vi "NI VeriStand - Search for Item by Property.vi"(8 "error in":errorcluster, 9 "Property Value":variant, 10 "Property Name":string, 11 "Section Ref in":T1 format="%.0x") -> (0 "error out":errorcluster, 2 "Item Ref":T1 format="%.0x", 3 "Section Ref out":T1 format="%.0x", 4 "Found":bool)   [LabVIEW 2020, in "Custom Device Utility Library.lvlib"]
doc: "Searches a custom device section for the item(s) you specify. You can search for one or multiple items by name, GUID, or property name and value. You must manually select the polymorphic instance to use."
uses:
  <vilib>/NI VeriStand/Custom Device Tools/Custom Device Utility Library/Custom Device Utility Library.lvlib
  <vilib>/NI VeriStand/Custom Device API/Custom Device Item Ref.ctl
  <vilib>/NI VeriStand/Custom Device Tools/Custom Device Utility Library/NI VeriStand - Ref Constants.vi
  <vilib>/NI VeriStand/Custom Device API/Get Item Property (Variant).vi
  <vilib>/NI VeriStand/Custom Device API/Custom Device API.lvlib
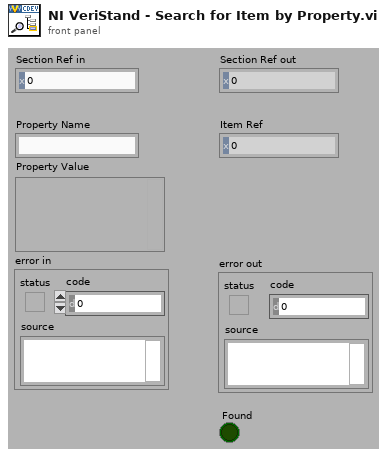
[diagram p1: front panel]
types:
  T1 = typedef "Custom Device API.lvlib/Custom Device Item Ref.ctl" = u64
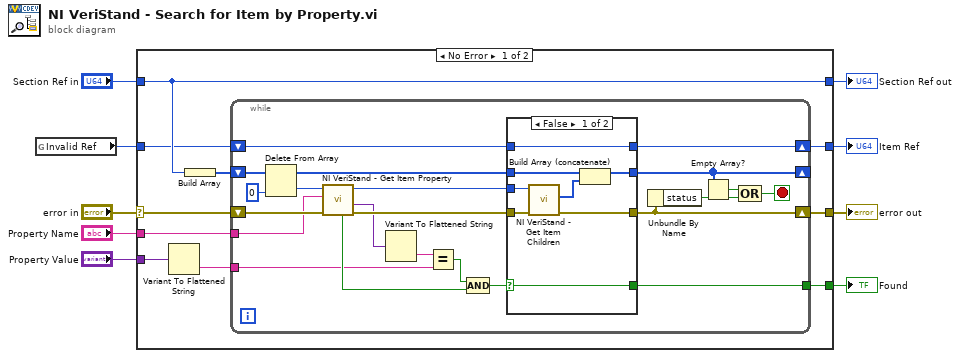
[diagram p0: block diagram]
diagram:
  n1 = global read "NI VeriStand - Ref Constants.vi" "Invalid Ref"() -> (w2:T1)
  n2 = case shown="No Error" "error in" {
    selector: "error in" -> [w14 w54]
    tunnel: "Section Ref in" -> [w15 w55]
    tunnel: "Property Name" -> [w18 _]
    tunnel: [w17 w54] -> w7
    tunnel: [w16 _] -> w6
    tunnel: [w13 w53] -> w5
    tunnel: [w15 w55] -> w4
    tunnel: w2 -> [w12 w53]
    tunnel: "Property Value" -> [w11 _]
    frame No Error {
      n3 = Variant To Flattened String(Variant=w11) -> (data string=w10:string)  [unwired: 1 out]
      n4 = Build Array(w15) -> (w19:T1[])
      n5 = while {
        shift-right: [w28] -> w17
        shift-left: w14 -> [w40]
        shift-right: [w27] -> _
        shift-left: w19 -> [w39]
        tunnel: w18 -> [w26]
        tunnel: [w33] -> w16
        shift-right: [w34] -> w13
        shift-left: w12 -> [w32]
        tunnel: w10 -> [w23]
        stop <- w29 stop-if-true
        n6 = Delete From Array(array=w39, index=0) -> (deleted portion=w37:T1, array with subset deleted=w35:T1[])  [unwired: 1 in]
        n7 = call-poly <vilib>:"NI VeriStand - Get Item Property.vi"("error in (no error)"=w40, "Property Name"=w26, "Item Ref in"=w37) -> ("error out"=w41:errorcluster, "Value"=w21:variant, "Item Ref out"=w36:T1, "Found?"=w25:bool)  [unwired: 1 in, 4 out]
        n8 = Variant To Flattened String(Variant=w21) -> (data string=w20:string)  [unwired: 1 out]
        n9 = Equal?(x=w20, y=w23) -> (x = y?=w22:bool)
        n10 = Compound Arithmetic op=AND(w22, w25) -> (w24:bool)
        n11 = case shown="False" w24 {
          selector: w24 -> [w43 w51]
          tunnel: [w49 w52] -> w28
          tunnel: w41 -> [w48 w52]
          tunnel: w36 -> [w47 w50]
          tunnel: w35 -> [w46 _]
          tunnel: [w44 _] -> w27
          tunnel: [w42 w50] -> w34
          tunnel: [w43 w51] -> w33
          tunnel: w32 -> [w42 _]
          frame False {
            n12 = call <vilib>:"NI VeriStand - Get Item Children.vi"("error in (no error)"=w48, "Item Ref in"=w47) -> ("error out"=w49:errorcluster, "Child Refs"=w45:T1[])  [unwired: 8 out]
            n13 = Build Array (concatenate)(w46, w45) -> (w44:T1[])
          }
          frame True {
          }
        }
        n14 = Unbundle By Name(w28) -> ("status"=w30:bool)
        n15 = Empty Array?(array=w27) -> (empty?=w31:bool)
        n16 = Compound Arithmetic op=OR(w31, w30) -> (w29:bool)
      }
    }
    frame Error {
    }
  }
  "Found" <- w6
  "error out" <- w7
  "Section Ref out" <- w4
  "Item Ref" <- w5
